vi "Sub-VI 2.vi"(0 "B1":bool, 1 "B2":bool, 2 "B3":bool, 3 "B4":bool, 4 "B5":bool, 5 "B6":bool, 6 "B7":bool, 7 "B8":bool, 8 "B9":bool, 10 "B10":bool, 12 "B11":bool, 16 "Chord name ?":bool, 18 "Stop conversion":bool, 20 "N1":bool, 21 "N2":bool, 22 "N3":bool, 23 "N4":bool, 24 "N5":bool, 25 "N6":bool, 26 "N7":bool, 27 "N8":bool) -> (15 "CORRESPONDING CHORD":string)   [LabVIEW 2019]
panel:
  out "Generated note ID":i16
  # "Welcome \ndear apprentices"
  # "This App, tailor-made for you, has magic power. Which ?  \nThat of making you travel in the shoes \nof one of the greatest pianists of all time :"
  # "Sir Elton John."
  # "Let yourself \nbe transported by its chords !"
  # "NOTE BOX"
  # "CHORD NAME BOX"
  # "1"
  # "2"
  # "3"
  # "4"
  # "5"
  # "6"
  # "7"
  # "8"
  # "3"
  # "4"
  # "5"
  # "6"
  # "8"
  # "9"
  # "10"
  # "1"
  # "2"
  # "7"
  # "11"
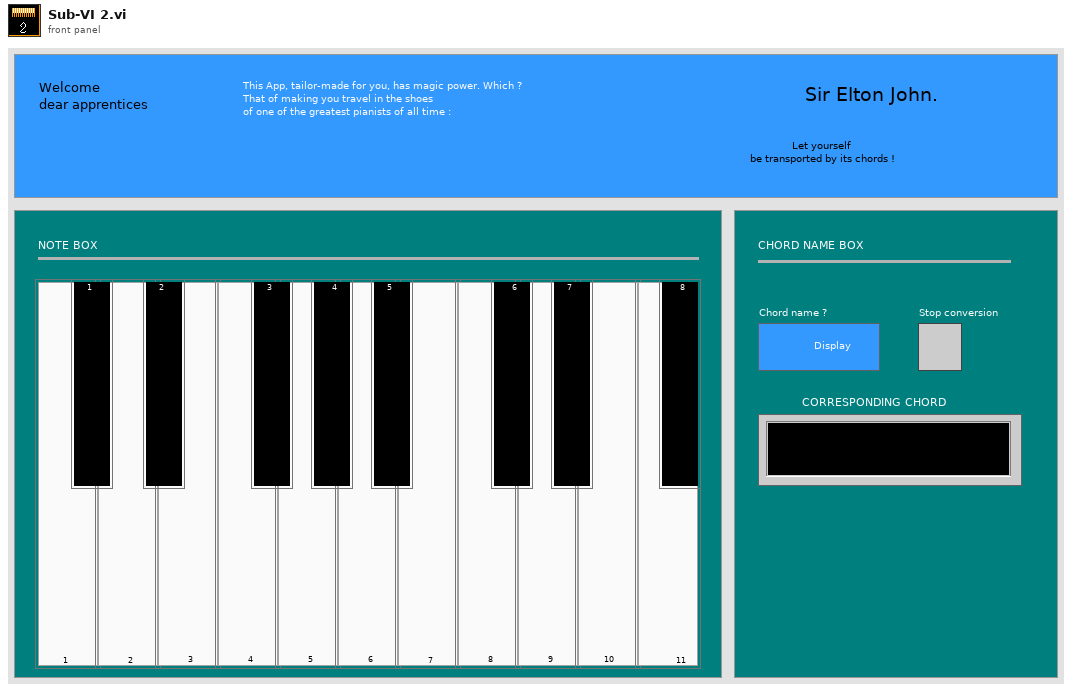
[diagram p1: front panel]
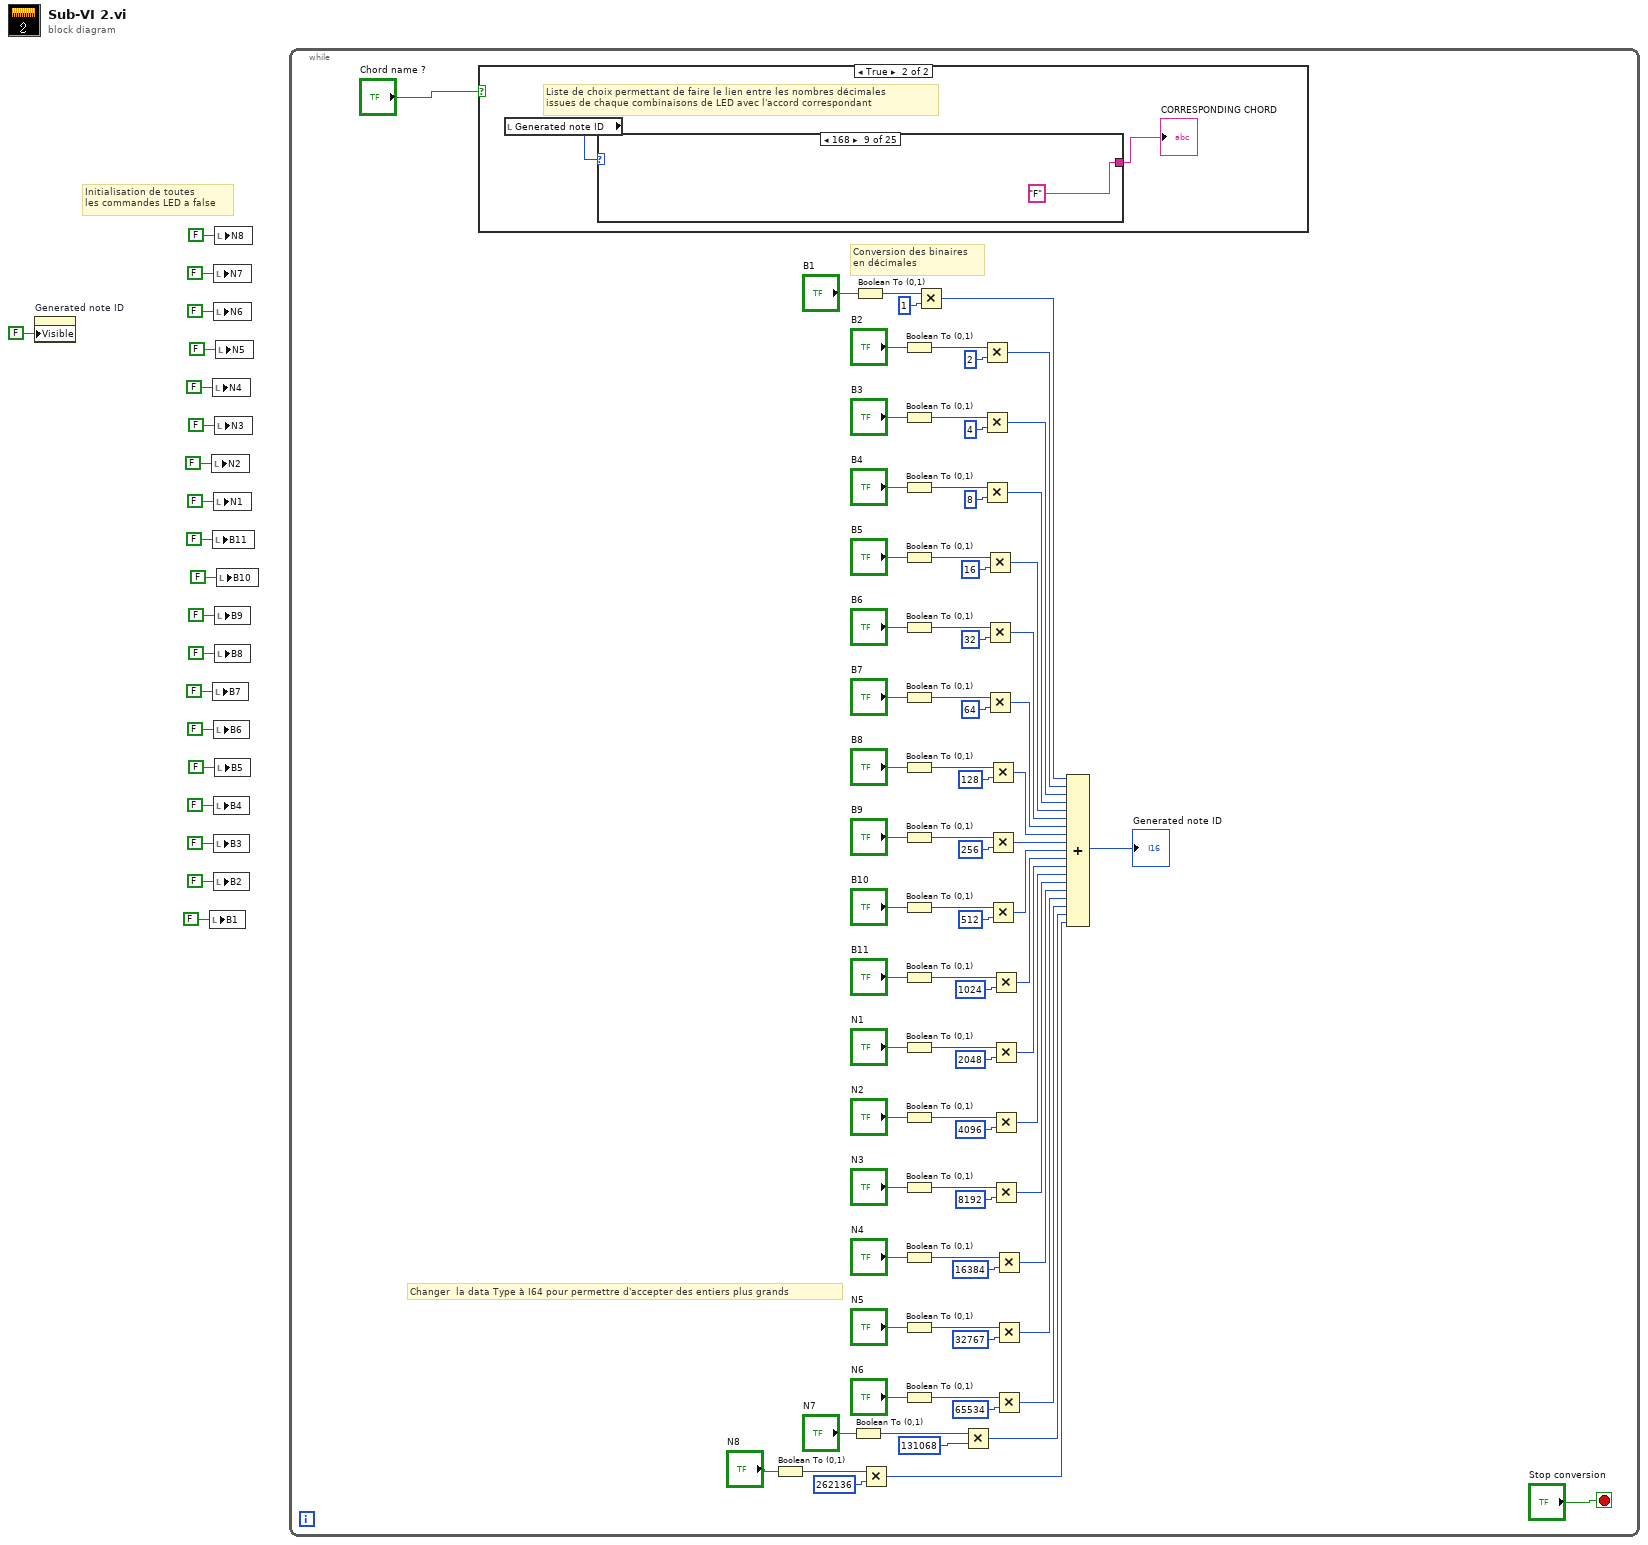
[diagram p0: block diagram]
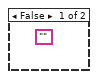
[diagram p2: hidden frame]
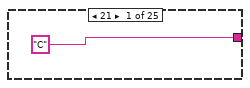
[diagram p3: hidden frame]
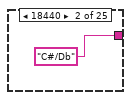
[diagram p4: hidden frame]
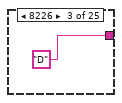
[diagram p5: hidden frame]
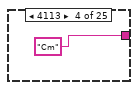
[diagram p6: hidden frame]
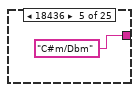
[diagram p7: hidden frame]
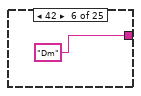
[diagram p8: hidden frame]
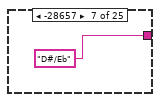
[diagram p9: hidden frame]
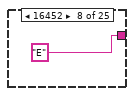
[diagram p10: hidden frame]
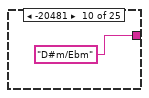
[diagram p11: hidden frame]
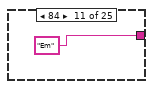
[diagram p12: hidden frame]
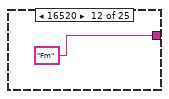
[diagram p13: hidden frame]
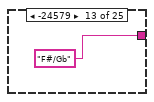
[diagram p14: hidden frame]
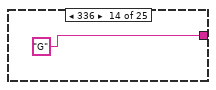
[diagram p15: hidden frame]
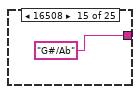
[diagram p16: hidden frame]
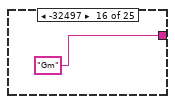
[diagram p17: hidden frame]
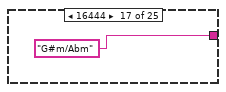
[diagram p18: hidden frame]
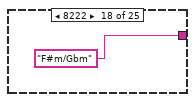
[diagram p19: hidden frame]
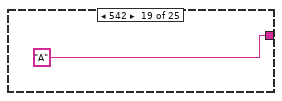
[diagram p20: hidden frame]
diagram:
  # "Initialisation de toutes\nles commandes LED a false"
  n1 = property on="Generated note ID" class="DigNum (strict)"("Visible"=FALSE) -> ()  [unwired: 2 in, 2 out]
  n2 = local write "B1"(FALSE) -> ()
  n3 = local write "N2"(FALSE) -> ()
  n4 = local write "N4"(FALSE) -> ()
  n5 = local write "B11"(FALSE) -> ()
  n6 = local write "B7"(FALSE) -> ()
  n7 = local write "N7"(FALSE) -> ()
  n8 = local write "N6"(FALSE) -> ()
  n9 = local write "N1"(FALSE) -> ()
  n10 = local write "B6"(FALSE) -> ()
  n11 = local write "B4"(FALSE) -> ()
  n12 = local write "B3"(FALSE) -> ()
  n13 = local write "B2"(FALSE) -> ()
  n14 = local write "N8"(FALSE) -> ()
  n15 = local write "N3"(FALSE) -> ()
  n16 = local write "B9"(FALSE) -> ()
  n17 = local write "B8"(FALSE) -> ()
  n18 = local write "B5"(FALSE) -> ()
  n19 = local write "N5"(FALSE) -> ()
  n20 = local write "B10"(FALSE) -> ()
  n21 = while {
    stop <- "Stop conversion" stop-if-true
    # "Changer  la data Type à I64 pour permettre d'accepter des entiers plus grands"
    # "Conversion des binaires\nen décimales"
    n22 = case shown="True" "Chord name ?" {
      frame False {
        (unwired) ""
      }
      frame True {
        # "Liste de choix permettant de faire le lien entre les nombres décimales \nissues de chaque combinaisons de LED avec l'accord correspondant"
        n23 = local read "Generated note ID"() -> (w100:i16)
        n24 = case shown="168" w100 {
          tunnel: ["C" "C#/Db" "D" "Cm" "C#m/Dbm" "Dm" "D#/Eb" "E" "F" "D#m/Ebm" "Em" "Fm" "F#/Gb" "G" "G#/Ab" "Gm" "G#m/Abm" "F#m/Gbm" "A" "A#/Bb" "B" "Am" "A#m/Bbm" "Bm" "You have selected an invalid combination of notes. Try again and please enter a correct note"] -> w101
          frame 21 {
          }
          frame 18440 {
          }
          frame 8226 {
          }
          frame 4113 {
          }
          frame 18436 {
          }
          frame 42 {
          }
          frame -28657 {
          }
          frame 16452 {
          }
          frame 168 {
          }
          frame -20481 {
          }
          frame 84 {
          }
          frame 16520 {
          }
          frame -24579 {
          }
          frame 336 {
          }
          frame 16508 {
          }
          frame -32497 {
          }
          frame 16444 {
          }
          frame 8222 {
          }
          frame 542 {
          }
          frame -31489 {
          }
          frame 52 {
          }
          frame 672 {
          }
          frame -31747 {
          }
          frame 312 {
          }
          frame 0, Default {
          }
        }
        "CORRESPONDING CHORD" <- w101
      }
    }
    n25 = Boolean To (0,1)(Boolean="N8") -> (0, 1=w56:i16)
    n26 = Boolean To (0,1)(Boolean="N7") -> (0, 1=w58:i16)
    n27 = Boolean To (0,1)(Boolean="B1") -> (0, 1=w98:i16)
    n28 = Multiply(x=w56, y=262136) -> (x*y=w24:i32)
    n29 = Boolean To (0,1)(Boolean="B2") -> (0, 1=w96:i16)
    n30 = Boolean To (0,1)(Boolean="B3") -> (0, 1=w94:i16)
    n31 = Boolean To (0,1)(Boolean="B4") -> (0, 1=w92:i16)
    n32 = Boolean To (0,1)(Boolean="B5") -> (0, 1=w84:i16)
    n33 = Boolean To (0,1)(Boolean="B6") -> (0, 1=w82:i16)
    n34 = Boolean To (0,1)(Boolean="B7") -> (0, 1=w80:i16)
    n35 = Boolean To (0,1)(Boolean="B8") -> (0, 1=w78:i16)
    n36 = Boolean To (0,1)(Boolean="B9") -> (0, 1=w76:i16)
    n37 = Boolean To (0,1)(Boolean="B10") -> (0, 1=w74:i16)
    n38 = Boolean To (0,1)(Boolean="B11") -> (0, 1=w72:i16)
    n39 = Boolean To (0,1)(Boolean="N1") -> (0, 1=w70:i16)
    n40 = Boolean To (0,1)(Boolean="N2") -> (0, 1=w68:i16)
    n41 = Boolean To (0,1)(Boolean="N3") -> (0, 1=w66:i16)
    n42 = Boolean To (0,1)(Boolean="N4") -> (0, 1=w64:i16)
    n43 = Boolean To (0,1)(Boolean="N5") -> (0, 1=w62:i16)
    n44 = Boolean To (0,1)(Boolean="N6") -> (0, 1=w60:i16)
    n45 = Multiply(x=w98, y=1) -> (x*y=w42:i32)
    n46 = Multiply(x=w58, y=131068) -> (x*y=w25:i32)
    n47 = Multiply(x=w96, y=2) -> (x*y=w41:i32)
    n48 = Multiply(x=w94, y=4) -> (x*y=w40:i32)
    n49 = Multiply(x=w92, y=8) -> (x*y=w39:i32)
    n50 = Multiply(x=w84, y=16) -> (x*y=w38:i32)
    n51 = Multiply(x=w82, y=32) -> (x*y=w37:i32)
    n52 = Multiply(x=w80, y=64) -> (x*y=w36:i32)
    n53 = Multiply(x=w78, y=128) -> (x*y=w35:i32)
    n54 = Multiply(x=w76, y=256) -> (x*y=w34:i32)
    n55 = Multiply(x=w74, y=512) -> (x*y=w33:i32)
    n56 = Multiply(x=w72, y=1024) -> (x*y=w32:i32)
    n57 = Multiply(x=w70, y=2048) -> (x*y=w31:i32)
    n58 = Multiply(x=w68, y=4096) -> (x*y=w30:i32)
    n59 = Multiply(x=w66, y=8192) -> (x*y=w29:i32)
    n60 = Multiply(x=w64, y=16384) -> (x*y=w28:i32)
    n61 = Multiply(x=w62, y=32767) -> (x*y=w27:i32)
    n62 = Multiply(x=w60, y=65534) -> (x*y=w26:i32)
    n63 = Compound Arithmetic op=ADD(w42, w41, w40, w39, w38, w37, w36, w35, w34, w33, w32, w31, w30, w29, w28, w27, w26, w25, w24) -> (→"Generated note ID":i32)
  }
